vi "PQexecPrepared.vi"(0 "stmtName":string, 1 "conn":u64, 5 "nParams":u64, 7 "paramValues":string[](array[string]), 9 "paramLengths":u64[](array[numeric]), 11 "paramFormats":u64[](array[numeric]), 12 "resultFormat":i64, 13 "error in (no error)":errorcluster) -> (4 "conn_out":u64, 8 "res":u64, 15 "error out":errorcluster)   [LabVIEW 2019, in "libpqlv64.lvlib"]
doc: "Sends a request to execute a prepared statement with given parameters, and waits for the result.\n\nhttp://www.postgresql.org/docs/8.1/interactive/libpq-exec.html"
uses:
  libpqlv64.lvlib
  libpq.dll
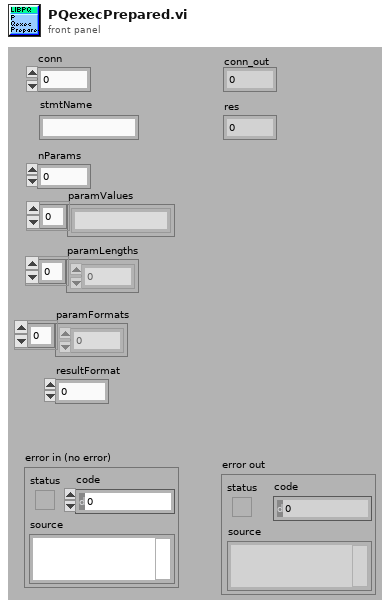
[diagram p1: front panel]
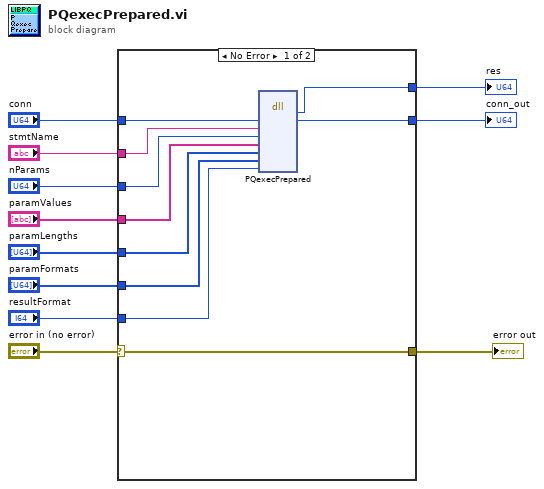
[diagram p0: block diagram]
diagram:
  n1 = case shown="No Error" "error in (no error)" {
    selector: "error in (no error)" -> [w21 w23]
    tunnel: [w21 w23] -> w10
    tunnel: [w20 _] -> w9
    tunnel: "stmtName" -> [w19 _]
    tunnel: "nParams" -> [w18 _]
    tunnel: "paramValues" -> [w17 _]
    tunnel: "paramLengths" -> [w16 _]
    tunnel: "paramFormats" -> [w15 _]
    tunnel: "resultFormat" -> [w14 _]
    tunnel: "conn" -> [w13 w22]
    tunnel: [w12 w22] -> w1
    frame No Error {
      n2 = dll-call lib="libpq.*" fn="PQexecPrepared"("conn"=w13, "stmtName"=w19, "nParams"=w18, "paramValues"=w17, "paramLengths"=w16, "paramFormats"=w15, "resultFormat"=w14) -> ("res"=w20:u64, "conn"=w12:u64)  [unwired: 9 in, 2 out]
    }
    frame Error {
    }
  }
  "res" <- w9
  "error out" <- w10
  "conn_out" <- w1
